vi "Gear Delivery SS Safety.vi"(11 "Gear Delivery Actuator In":T1={"Gear Release"=enum."Reverse", "Gear Intake"=enum."Off", "Gear Chute"=enum."Off"}) -> (3 "Gear Delivery Actuator Out":T1={"Gear Release"=enum."Reverse", "Gear Intake"=enum."Off", "Gear Chute"=enum."Off"})   [LabVIEW 2016]
uses:
  Gear Delivery Actuator Out.ctl
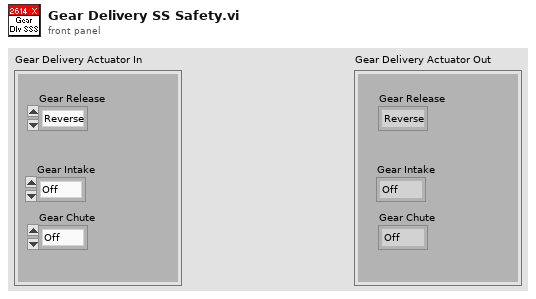
[diagram p1: front panel]
types:
  T1 = typedef "Gear Delivery Actuator Out.ctl" = cluster{"Gear Release":enum16{"Off", "On", "Forward", "Reverse"}, "Gear Intake":enum16{"Off", "On", "Forward", "Reverse"}, "Gear Chute":enum16{"Off", "On", "Forward", "Reverse"}}
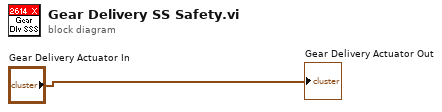
[diagram p0: block diagram]
diagram:
  "Gear Delivery Actuator Out" <- "Gear Delivery Actuator In"
